vi "Send To Recievers.vi"(8 "error in (no error)":errorcluster, 9 "priority":T1, 10 "Message":refnum<class "Message.lvclass">, 11 "Pub Sub Message Channel in":refnum<class "Pub Sub Message Channel.lvclass">) -> (0 "error out":errorcluster)   [LabVIEW 2020, in "Actor Pub Sub Channels.lvlib" / "Pub Sub Message Channel.lvclass"]
uses:
  Pub Sub Message Channel.lvclass
  <vilib>/ActorFramework/Message/Message.lvclass
  <vilib>/ActorFramework/Message Dequeuer/Dequeue Priority.ctl
  Pub Sub Message Channel.lvclass/Pub Sub Message Channel.ctl
  <vilib>/ActorFramework/Self-Addressed Msg/Self-Addressed Msg.lvclass/Self-Addressed Msg.ctl
  <vilib>/ActorFramework/Message Enqueuer/Message Enqueuer.lvclass
  <vilib>/ActorFramework/Self-Addressed Msg/Self-Addressed Msg.lvclass
  <vilib>/ActorFramework/Message Dequeuer/Message Dequeuer.lvclass
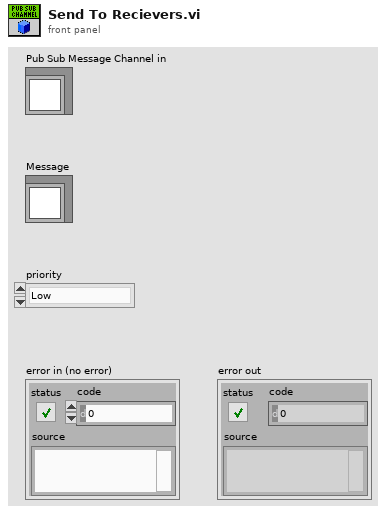
[diagram p1: front panel]
types:
  T1 = typedef "Actor Framework.lvlib/Message Dequeuer.lvclass/Dequeue Priority.ctl" = enum16{"Low", "Normal", "High", "Critical"}
  T2 = map{refnum<class "Message Enqueuer.lvclass">, string}
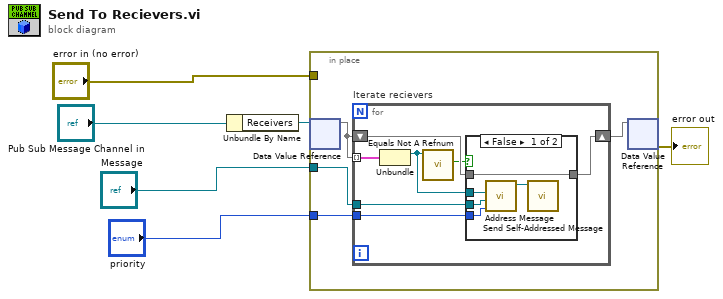
[diagram p0: block diagram]
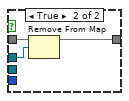
[diagram p2: hidden frame]
diagram:
  n1 = Unbundle By Name("Pub Sub Message Channel in") -> ("Receivers"=w3:refnum<data-value>)
  n2 = in-place {
    in-place-border: "Message" -> [w10]
    in-place-border: "priority" -> [w9]
    in-place-border: "error in (no error)" -> [_]
    n3 = in-place-dvr #1(w3) -> (w8:T2)  [unwired: 1 out]
    n4 = for "Iterate recievers" {
      tunnel: w8 -> [w17] mode=indexing
      tunnel: w10 -> [w12]
      tunnel: w9 -> [w13]
      shift-right: [w15] -> w7
      shift-left: w8 -> [w16]
      n5 = Unbundle(w17) -> ("Message Enqueuer"=w11:refnum<class "Message Enqueuer.lvclass">)  [unwired: 1 out]
      n6 = call <vilib>:"Equals Not A Refnum.vi"("Message Enqueuer"=w11) -> ("Not a refnum?"=w14:bool)  [unwired: 10 in]
      n7 = case shown="False" w14 {
        tunnel: w16 -> [w18 w25]
        tunnel: [w18 w24] -> w15
        tunnel: w11 -> [w19 w23]
        tunnel: w13 -> [w22 _]
        tunnel: w12 -> [w21 _]
        frame False {
          n8 = call <vilib>:"Address Message.vi"("Message Priority (Normal)"=w22, "Message"=w21, "Destination"=w19) -> ("Self-Addressed Message"=w20:refnum<class "Self-Addressed Msg.lvclass">)  [unwired: 8 in]
          n9 = call-dynamic "Send Self-Addressed Message.vi"("Self-Addressed Message in"=w20) -> ()  [unwired: 9 in, 2 out]
        }
        frame True {
          n10 = Remove From Map(10:w23, 11:w25) -> (3:w24:T2)  [unwired: 2 out]
        }
      }
    }
    n11 = in-place-dvr #1(w7) -> (→"error out":errorcluster)  [unwired: 1 out]
  }
